vi "CRYWrite Harmonics list file.vi"(11 "Harmonics list":string[](array[string])) -> ()   [LabVIEW 2013]
uses:
  CRYMainGlobal.vi
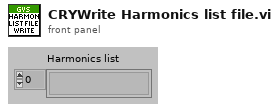
[diagram p1: front panel]
types:
  T1 = enum16{"open", "open or create", "create or replace", "create"}
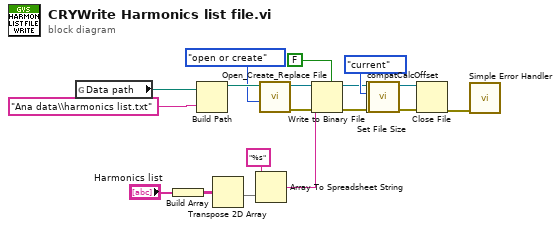
[diagram p0: block diagram]
diagram:
  n1 = global read "CRYMainGlobal.vi" "Data path"() -> (w1:path)
  n2 = Build Array("Harmonics list") -> (w20:string[][])
  n3 = Build Path(base path=w1, name or relative path="Ana data\\harmonics list.txt") -> (appended path=w8:path)
  n4 = Transpose 2D Array(2D array=w20) -> (transposed array=w19:string[][])
  n5 = Array To Spreadsheet String(array=w19, 3:"%s" ("format string")) -> (spreadsheet string=w17:string)  [unwired: 1 out]
  n6 = call <vilib>:"Open_Create_Replace File.vi"("function (open:0)"=T1."open or create", "file path"=w8) -> ("error out"=w9:errorcluster, "refnum"=w10:refnum<file>)  [unwired: 4 in, 4 out]
  n7 = Write to Binary File(file (use dialog)=w10, data=w17, error in=w9, 5:FALSE ("预置数组或字符串大小？(T)")) -> (refnum out=w15:refnum<file>, error out=w14:errorcluster)  [unwired: 3 out]
  n8 = call <vilib>:"compatCalcOffset.vi"("error in"=w14, "pos mode (0:1)"=enum16{"start", "end", "current"}."current", "refnum"=w15) -> ("error out"=w6:errorcluster, "offset"=w5:i32, "dup refnum"=w4:refnum<file>)  [unwired: 1 in, 5 out]
  n9 = Set File Size(4:w6, 6:w5, 7:w4) -> (0:w12:errorcluster, 3:w11:refnum<file>)
  n10 = Close File(refnum=w11, error in=w12) -> (error out=w13:errorcluster)  [unwired: 1 out]
  n11 = call <vilib>:"Simple Error Handler.vi"("error in (no error)"=w13) -> ()  [unwired: 1 in, 8 out]
